vi "Yannick.vi"(9 "REPL":string, 10 "Send":string) -> ()   [LabVIEW 2020]
uses:
  <vilib>/Instr/_visa.llb/VISA Configure Serial Port (Instr).vi
panel:
  in  "Board":string="Arduino Nano 33 IoT"
  out "Cover":bool
  in  "Script":string
  in  "Buffer":string
  in  "Disconnect":bool
  in  "Help":bool
  in  "Connect":bool
  in  "Stop Button":bool
  in  "Port":refnum<visa-resource-name>
  out "Running Script":bool
  in  "Abort":bool
  in  "xPort":string
  # "MAC ONLY"
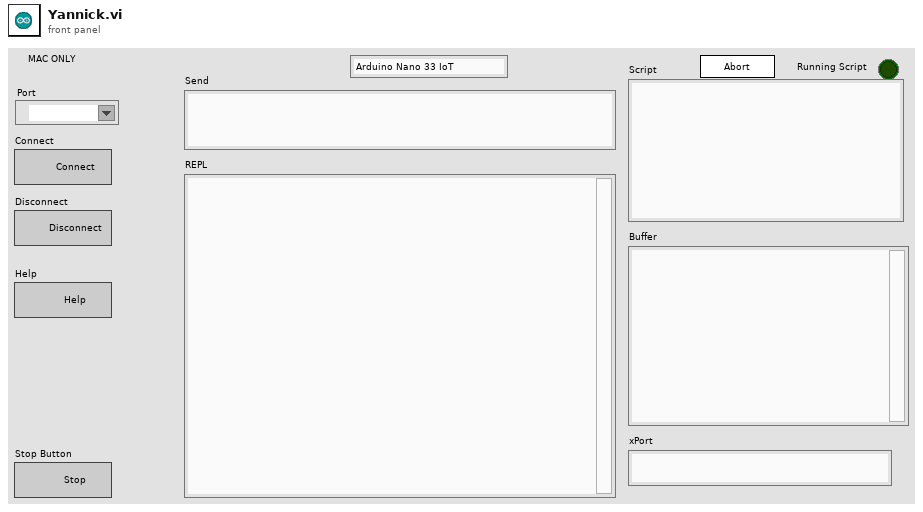
[diagram p1: front panel]
types:
  T1 = enum32{"Invalid", "Standard", "Closed", "Hidden", "Minimized", "Maximized"}
  T2 = typedef "eventvkey.ctl" = enum16{"ASCII", "Enter", "Return", "Shift", "Ctrl", "Alt", "Cmd", "Opt", "Caps", "NumLock", "Clear", "Break", "Up", "Down", "Left", "Right", "Insert", "Delete", "Home", "End", "PageUp", "PageDown", "Escape", "Help", "Pause", "ScrollLock", "F1", "F2", "F3", "F4", "F5", "F6", "F7", "F8", "F9", "F10", "F11", "F12", "F13", "F14", "F15", "F16", "F17", "F18", "F19", "F20", "F21", "F22", "F23", "F24", "Play", "VolumeUp", "VolumeDown", "Mute", "Two Byte Char"}
  T3 = cluster{"Shift":bool, "Ctrl":bool, "Alt":bool, "Cmd":bool, "Opt":bool}
  T4 = cluster{"Char":i16, "VKey":T2, "PlatMods":cluster{"Shift":bool, "Ctrl":bool, "Alt":bool, "Cmd":bool, "Opt":bool}}
  T5 = typedef "Arduino.ctl" = cluster{"Java":path, "Packages":path, "folder":path, "serial":string, "Console":string}
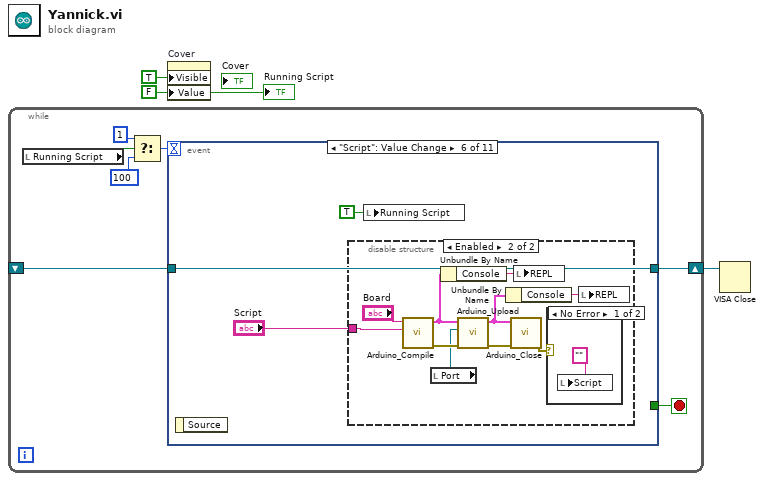
[diagram p0: block diagram]
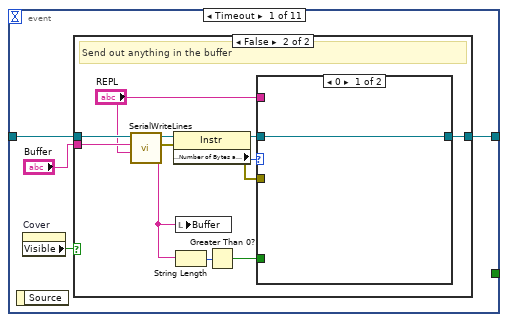
[diagram p2: hidden frame]
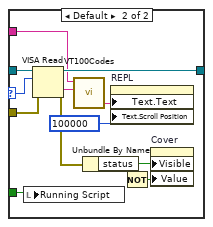
[diagram p4: hidden frame]
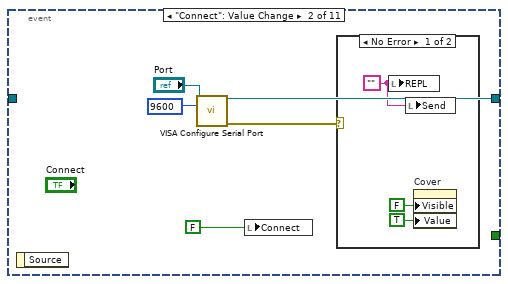
[diagram p5: hidden frame]
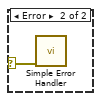
[diagram p6: hidden frame]
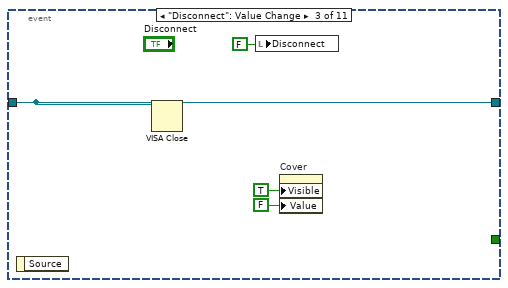
[diagram p7: hidden frame]
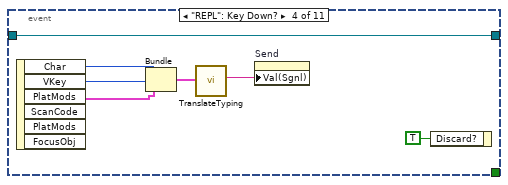
[diagram p8: hidden frame]
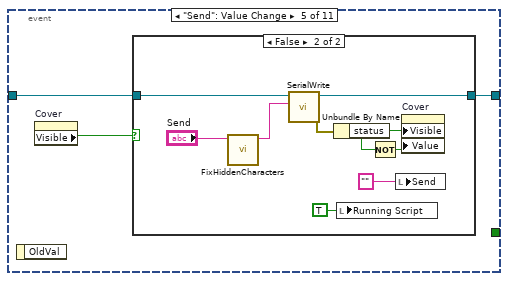
[diagram p9: hidden frame]
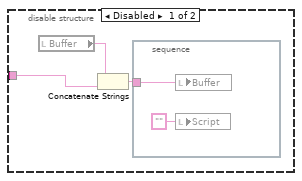
[diagram p11: hidden frame]
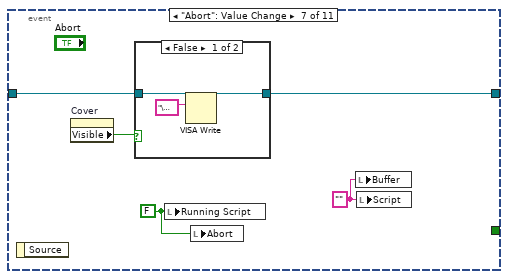
[diagram p13: hidden frame]
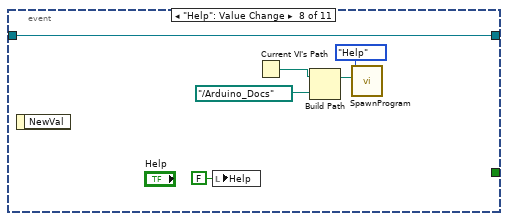
[diagram p15: hidden frame]
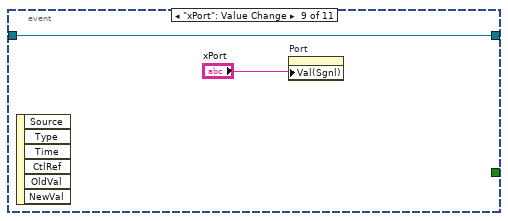
[diagram p16: hidden frame]
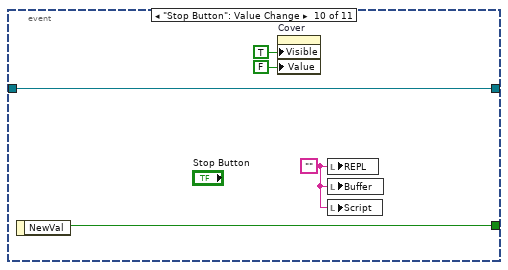
[diagram p17: hidden frame]
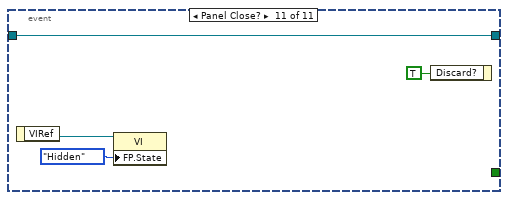
[diagram p18: hidden frame]
diagram:
  w1 = FALSE ("Cover")
  n1 = while {
    shift-right: [w9] -> w2
    shift-left: _ -> [w8]
    stop <- w10 stop-if-true
    n2 = local read "Running Script"() -> (w4:bool)
    n3 = Select(t=1, s=w4, f=100) -> (s? t:f=w5:i32)
    n4 = event shown="[5] \"Script\": Value Change" {
      selector: _ -> [_ _ _ _ _ _ _ _ _ _ _]
      dyn-events: _ -> [_ _ _ _ _ _ _ _ _ _ _]
      timeout: w5 -> [_ _ _ _ _ _ _ _ _ _ _]
      tunnel: [_ _ _ _ _ _ _ _ _ w112 _] -> w10
      tunnel: [w14 w41 w52 w59 w61 w75 w95 w106 w108 w113 w117] -> w9
      tunnel: w8 -> [w13 _ w52 w59 w62 w75 w94 w106 w108 w113 w117]
      event Timeout {
        n5 = event-data() -> ()  [unwired: 1 in, 1 out]
        n6 = property on="Cover" class="Bool (strict)"() -> ("Visible"=w12:bool)  [unwired: 2 in, 2 out]
        n7 = case shown="False" w12 {
          tunnel: [w15 w26] -> w14
          tunnel: w13 -> [w15 w25]
          tunnel: "Buffer" -> [_ w24]
          frame True {
          }
          frame False {
            # "Send out anything in the buffer"
            n8 = call "SerialWriteLines.vi"("REPL"="REPL", "Send"=w24, "VISA Refnum in"=w25) -> ("error out"=w21:errorcluster, "Rest"=w18:string, "VISA Refnum out"=w23:refnum<visa-resource-name>)  [unwired: 6 in]
            n9 = property class="Instr"(reference=w23, error in=w21) -> (error out=w20:errorcluster, "Serial Settings:Number of Bytes at Serial Port"=w22:u32)  [unwired: 1 out]
            n10 = local write "Buffer"(w18) -> ()
            n11 = String Length(string=w18) -> (length=w19:i32)
            n12 = Greater Than 0?(x=w19) -> (x > 0?=w17:bool)
            n13 = case shown="0" w22 {
              selector: w22 -> [_ w35]
              tunnel: [w27 w39] -> w26
              tunnel: w23 -> [w27 w38]
              tunnel: w20 -> [_ w33]
              tunnel: w17 -> [_ w31]
              tunnel: "REPL" -> [_ w30]
              frame 0 {
              }
              frame Default {
                n14 = local write "Running Script"(w31) -> ()
                n15 = VISA Read(VISA resource name=w38, byte count=w35, error in (no error)=w33) -> (VISA resource name out=w39:refnum<visa-resource-name>, read buffer=w36:string, error out=w32:errorcluster)  [unwired: 1 out]
                n16 = call "VT100Codes.vi"("read buffer"=w36, "Console In"=w30) -> ("Console Out"=w34:string)  [unwired: 9 in]
                n17 = Unbundle By Name(w32) -> ("status"=w28:bool)
                n18 = property on="REPL" class="Str"("Text.Text"=w34, "Text.Scroll Position"=u32 100000 ("Text.Selection:Start")) -> ()  [unwired: 2 in, 2 out]
                n19 = Not(x=w28) -> (.not. x?=w29:bool)
                n20 = property on="Cover" class="Bool (strict)"("Visible"=w28, "Value"=w29) -> ()  [unwired: 2 in, 2 out]
              }
            }
          }
        }
      }
      event "Connect": Value Change {
        n21 = event-data() -> ()  [unwired: 1 in, 1 out]
        n22 = call-poly "VISA Configure Serial Port"("VISA resource name"="Port", "baud rate (9600)"=u32 9600) -> ("VISA resource name out"=w41:refnum<visa-resource-name>, "error out"=w40:errorcluster)  [unwired: 12 in]
        n23 = local write "Connect"(FALSE ("Help")) -> ()
        n24 = case shown="No Error" w40 {
          selector: w40 -> [_ w48]
          frame No Error {
            w47 = ""
            n25 = local write "REPL"(w47) -> ()
            n26 = local write "Send"(w47) -> ()
            n27 = property on="Cover" class="Bool (strict)"("Visible"=FALSE, "Value"=TRUE ("Cover")) -> ()  [unwired: 2 in, 2 out]
          }
          frame Error {
            n28 = call <vilib>:"Simple Error Handler.vi"("error in (no error)"=w48) -> ()  [unwired: 4 in, 5 out]
          }
        }
      }
      event "Disconnect": Value Change {
        n29 = event-data() -> ()  [unwired: 1 in, 1 out]
        n30 = VISA Close(VISA resource name=w52) -> ()  [unwired: 1 in, 1 out]
        n31 = local write "Disconnect"(FALSE ("Help")) -> ()
        n32 = property on="Cover" class="Bool (strict)"("Visible"=TRUE, "Value"=FALSE ("Cover")) -> ()  [unwired: 2 in, 2 out]
      }
      event "REPL": Key Down? {
        n33 = event-data() -> ("Char"=w55:i16, "VKey"=w56:T2, "PlatMods"=w57:T3)  [unwired: 1 in, 3 out]
        n34 = Bundle("Char"=w55, "VKey"=w56, "PlatMods"=w57) -> (w58:T4)  [unwired: 1 in]
        n35 = call "TranslateTyping.vi"("Cluster"=w58) -> ("key"=w54:string)  [unwired: 10 in]
        n36 = property on="Send" class="Str"("Val(Sgnl)"=w54) -> ()  [unwired: 2 in, 2 out]
        n37 = event-data("Discard?"=TRUE) -> ()  [unwired: 1 in, 1 out]
      }
      event "Send": Value Change {
        n38 = event-data() -> ()  [unwired: 1 in, 1 out]
        n39 = property on="Cover" class="Bool (strict)"() -> ("Visible"=w60:bool)  [unwired: 2 in, 2 out]
        n40 = case shown="False" w60 {
          tunnel: w62 -> [w63 w72]
          tunnel: [w63 w71] -> w61
          frame True {
          }
          frame False {
            n41 = call "FixHiddenCharacters.vi"("String in"="Send") -> ("String out"=w67:string)  [unwired: 10 in]
            n42 = call "SerialWrite.vi"("Text"=w67, "VISA Refnum in"=w72) -> ("error out"=w64:errorcluster, "VISA Refnum out"=w71:refnum<visa-resource-name>)  [unwired: 8 in]
            n43 = Unbundle By Name(w64) -> ("status"=w65:bool)
            n44 = local write "Running Script"(TRUE ("Running Script")) -> ()
            n45 = Not(x=w65) -> (.not. x?=w66:bool)
            n46 = local write "Send"("" ("Write text")) -> ()
            n47 = property on="Cover" class="Bool (strict)"("Visible"=w65, "Value"=w66) -> ()  [unwired: 2 in, 2 out]
          }
        }
      }
      event "Script": Value Change {
        n48 = event-data() -> ()  [unwired: 1 in, 1 out]
        n49 = disable-structure shown="Enabled" {
          disable-tunnel: "Script" -> [w76 w90]
          frame Disabled {
            n50 = local read "Buffer"() -> (w78:string)
            n51 = Concatenate Strings(w78, w76) -> (w77:string)
            n52 = stacked-sequence {
              tunnel: w77 -> [w80]
              frame #0 {
                n53 = local write "Buffer"(w80) -> ()
                n54 = local write "Script"("" ("Script")) -> ()
              }
            }
          }
          frame Enabled {
            n55 = call "Arduino_Compile.vi"("Code"=w90, "Board"="Board") -> ("error out"=w87:errorcluster, "Arduino Out"=w82:T5)  [unwired: 8 in]
            n56 = local read "Port"() -> (w86:refnum<visa-resource-name>)
            n57 = Unbundle By Name(w82) -> ("Console"=w83:string)
            n58 = call "Arduino_Upload.vi"("error in (no error)"=w87, "VISA resource name"=w86, "Arduino In"=w82) -> ("error out"=w88:errorcluster, "Arduino Out"=w85:T5)  [unwired: 7 in]
            n59 = Unbundle By Name(w85) -> ("Console"=w84:string)
            n60 = call "Arduino_Close.vi"("error in (no error)"=w88, "Arduino In"=w85) -> ("error out"=w81:errorcluster)  [unwired: 8 in, 1 out]
            n61 = local write "REPL"(w83) -> ()
            n62 = case shown="No Error" w81 {
              frame No Error {
                n63 = local write "Script"("") -> ()
              }
              frame Error {
              }
            }
            n64 = local write "REPL"(w84) -> ()
          }
        }
        n65 = local write "Running Script"(TRUE ("Visible")) -> ()
      }
      event "Abort": Value Change {
        w96 = "" ("Script")
        w93 = FALSE ("Visible")
        n66 = event-data() -> ()  [unwired: 1 in, 1 out]
        n67 = property on="Cover" class="Bool (strict)"() -> ("Visible"=w92:bool)  [unwired: 2 in, 2 out]
        n68 = case shown="False" w92 {
          tunnel: [w98 w100] -> w95
          tunnel: w94 -> [w97 w100]
          frame False {
            n69 = VISA Write(VISA resource name=w97, write buffer="\u0003") -> (VISA resource name out=w98:refnum<visa-resource-name>)  [unwired: 1 in, 2 out]
          }
          frame True {
          }
        }
        n70 = local write "Running Script"(w93) -> ()
        n71 = local write "Abort"(w93) -> ()
        n72 = local write "Buffer"(w96) -> ()
        n73 = local write "Script"(w96) -> ()
      }
      event "Help": Value Change {
        n74 = event-data() -> ()  [unwired: 1 in, 1 out]
        n75 = local write "Help"(FALSE ("Help")) -> ()
        n76 = Current VI's Path() -> (path=w104:path)
        n77 = Build Path(base path=w104, name or relative path=path "../Arduino_Docs") -> (appended path=w102:path)
        n78 = call "SpawnProgram.vi"("Server"=w102, "Dialog"=enum16{"Help", "Files"}."Help") -> ()  [unwired: 10 in]
      }
      event "xPort": Value Change {
        n79 = event-data() -> ()  [unwired: 1 in, 6 out]
        n80 = property on="Port" class="VISAName"("Val(Sgnl)"="xPort") -> ()  [unwired: 2 in, 2 out]
      }
      event "Stop Button": Value Change {
        w109 = ""
        n81 = event-data() -> ("NewVal"=w112:bool)  [unwired: 1 in]
        n82 = property on="Cover" class="Bool (strict)"("Visible"=TRUE, "Value"=FALSE ("Cover")) -> ()  [unwired: 2 in, 2 out]
        n83 = local write "REPL"(w109) -> ()
        n84 = local write "Buffer"(w109) -> ()
        n85 = local write "Script"(w109) -> ()
      }
      event Panel Close? {
        n86 = event-data() -> ("VIRef"=w115:refnum<vi>)  [unwired: 1 in]
        n87 = property class="VI"(reference=w115, "FP.State"=T1."Hidden" ("Front Panel Window:State")) -> ()  [unwired: 1 in, 2 out]
        n88 = event-data("Discard?"=TRUE) -> ()  [unwired: 1 in, 1 out]
      }
    }
  }
  n89 = property on="Cover" class="Bool (strict)"("Visible"=TRUE, "Value"=w1) -> ()  [unwired: 2 in, 2 out]
  n90 = VISA Close(VISA resource name=w2) -> ()  [unwired: 1 in, 1 out]
  "Running Script" <- w1
